vi "Next Step.vi"(8 "error in (no error)":errorcluster, 11 "Combined Measurement in":refnum<class "Combined Measurement.lvclass">) -> (0 "error out":errorcluster, 3 "Combined Measurement out":refnum<class "Combined Measurement.lvclass">)   [LabVIEW 2021, in "Combined Measurement.lvclass"]
uses:
  Combined Measurement.lvclass
  Combined Measurement.lvclass/Combined Measurement.ctl
  Measurements/Response Synchronizer/Response Synchronizer.lvclass
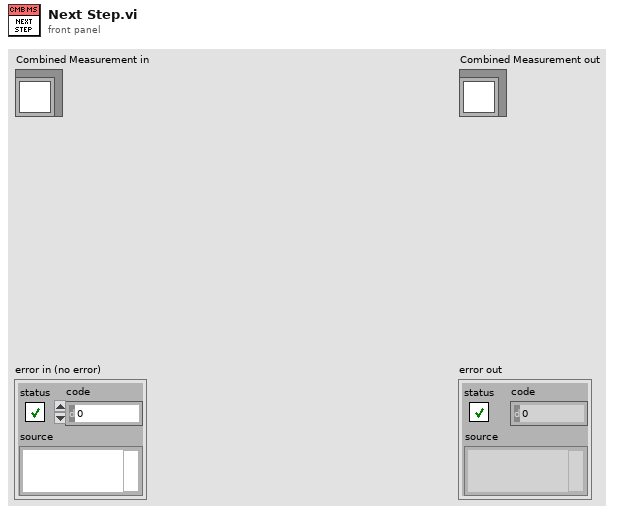
[diagram p1: front panel]
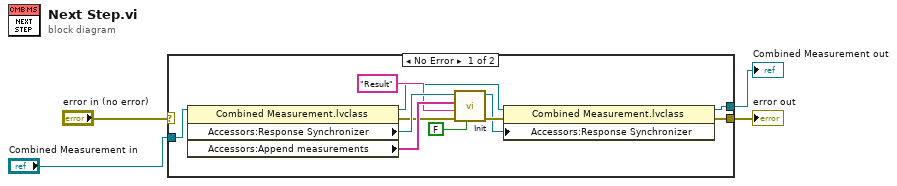
[diagram p0: block diagram]
diagram:
  n1 = case shown="No Error" "error in (no error)" {
    selector: "error in (no error)" -> [_ w17]
    tunnel: [w7 w17] -> w3
    tunnel: [w6 w16] -> w1
    tunnel: "Combined Measurement in" -> [w5 w16]
    frame No Error {
      n2 = property class="Combined Measurement.lvclass"(reference=w5) -> (reference out=w11:refnum<class "Combined Measurement.lvclass">, error out=w10:errorcluster, "Accessors:Response Synchronizer"=w15:refnum<class "Response Synchronizer.lvclass">, "Accessors:Append measurements"=w14:string[])  [unwired: 1 in]
      n3 = call-dynamic "Init.vi"("Subscribe"=FALSE, "error in (no error)"=w10, "Topic"="Result", "Responder names"=w14, "Response Synchronizer in"=w15) -> ("error out"=w9:errorcluster, "Response Synchronizer out"=w8:refnum<class "Response Synchronizer.lvclass">)  [unwired: 5 in]
      n4 = property class="Combined Measurement.lvclass"(reference=w11, error in=w9, "Accessors:Response Synchronizer"=w8) -> (reference out=w6:refnum<class "Combined Measurement.lvclass">, error out=w7:errorcluster)
    }
    frame Error {
    }
  }
  "error out" <- w3
  "Combined Measurement out" <- w1
